vi "Get Double By Name.vi"(0 "name":string, 2 "Analog Values":T1) -> (7 "result":dbl, 9 "found?":bool)   [LabVIEW 2011]
uses:
  Controls/Analog Values.ctl
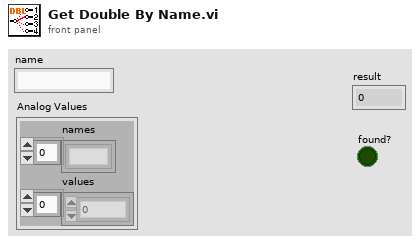
[diagram p1: front panel]
types:
  T1 = typedef "Analog Values.ctl" = cluster{"names":string[], "values":dbl[]}
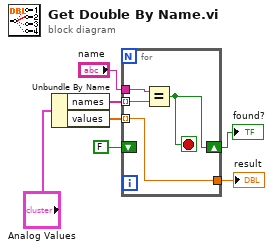
[diagram p0: block diagram]
diagram:
  n1 = Unbundle By Name("Analog Values") -> ("names"=w7:string[], "values"=w6:dbl[])
  n2 = for {
    tunnel: w7 -> [w9] mode=indexing
    tunnel: w6 -> [w11] mode=indexing
    tunnel: [w11] -> w1
    tunnel: "name" -> [w10]
    shift-right: [w8] -> w3
    shift-left: FALSE -> [_]
    stop <- w8 stop-if-true
    n3 = Equal?(x=w10, y=w9) -> (x = y?=w8:bool)
  }
  "found?" <- w3
  "result" <- w1
